vi "GetLastErrorCode.vi"(8 "error in":errorcluster, 11 "VISA resource name":refnum<visa-resource-name>) -> (0 "error out":errorcluster, 1 "Error Code":i32, 2 "Last error code":string, 3 "VISA resource name out":refnum<visa-resource-name>)   [LabVIEW 2023, in "Thermotron 8800.lvlib"]
doc: "IERR\nCommand name: Send last error code\nCommand type: System status\nDescription: The 8800 sends the code of the last error that occurred. For more information see\n“Error codes” later in this section.\nSyntax: IERR?\nData type: Coded integer\nQuery example: IERR?\n8800 response: 3 (The 8800 output buffer is full.)\nNOTE: The error code buffer holds the last eight errors. You can use the IERR? command\nrepeatedly to read the entire buffer in a first in–last out format. When the 8800 returns an error code of 0, the error buffer is empty."
uses:
  Thermotron 8800.lvlib
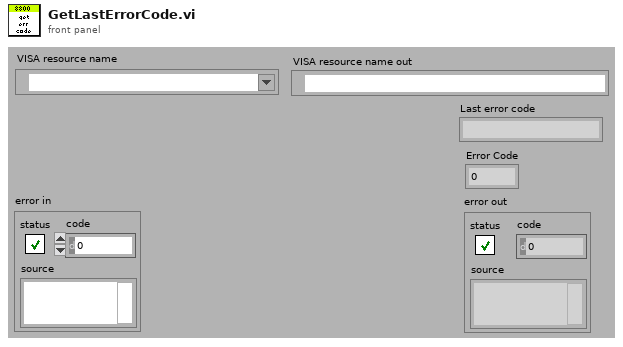
[diagram p1: front panel]
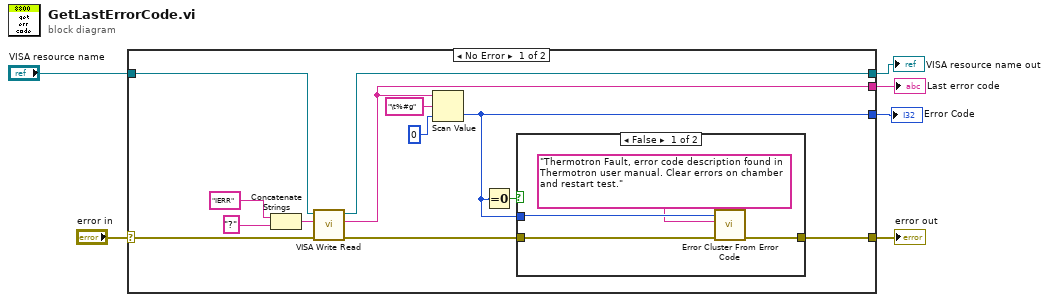
[diagram p0: block diagram]
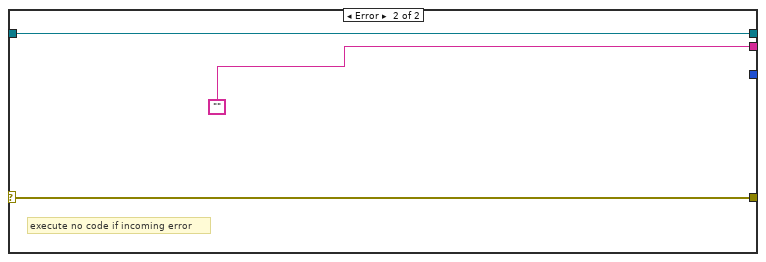
[diagram p3: hidden frame]
diagram:
  n1 = case shown="No Error" "error in" {
    selector: "error in" -> [w18 w27]
    tunnel: [w9 w27] -> w3
    tunnel: [w17 w25] -> w4
    tunnel: [w11 ""] -> w2
    tunnel: "VISA resource name" -> [w14 w25]
    tunnel: [w7 _] -> w1
    frame No Error {
      n2 = Concatenate Strings("IERR" ("8800 Command"), "?" ("8800 Command")) -> (w19:string)
      n3 = call "VISA Write Read.vi"("error in (no error)"=w18, "8800 Command"=w19, "VISA Refnum in"=w14) -> ("error out"=w10:errorcluster, "read buffer"=w11:string, "VISA Refnum out"=w17:refnum<visa-resource-name>)  [unwired: 6 in]
      n4 = Scan Value(string=w11, format string="\t%#g", default (0 dbl)=0) -> (value=w7:i32)  [unwired: 1 out]
      n5 = Equal To 0?(x=w7) -> (x = 0?=w8:bool)
      n6 = case shown="False" w8 {
        tunnel: w10 -> [w23 w24]
        tunnel: w7 -> [w22 _]
        tunnel: [w21 w24] -> w9
        frame False {
          n7 = call <vilib>:"Error Cluster From Error Code.vi"("error in (no error)"=w23, "error message (\"\")"="Thermotron Fault, error code description found in Thermotron user manual. Clear errors on chamber and restart test." ("error message (\"\")"), "error code (0)"=w22) -> ("error out"=w21:errorcluster)  [unwired: 6 in]
        }
        frame True {
        }
      }
    }
    frame Error {
      # "execute no code if incoming error"
    }
  }
  "VISA resource name out" <- w4
  "error out" <- w3
  "Last error code" <- w2
  "Error Code" <- w1
